vi "Start-Stop-Exp-Lock_UnLock.vi"(8 "entrée d'erreur (pas d'erreur)":errorcluster, 10 "Control-Client old entrée":refnum<class "Control-Client.lvclass">, 11 "Control-Client new entrée":refnum<class "Control-Client.lvclass">) -> (0 "sortie d'erreur":errorcluster, 2 "Control-Client old out":refnum<class "Control-Client.lvclass">, 3 "Control-Client new out":refnum<class "Control-Client.lvclass">)   [LabVIEW 2019, in "Control-Client.lvclass"]
uses:
  Control-Client.lvclass
  Control-Client.lvclass/Control-Client.ctl
  controls/Gauge_pump/Gauge_pump.xctl
  dependecies/XControls/CellsDL/ControlDL.xctl
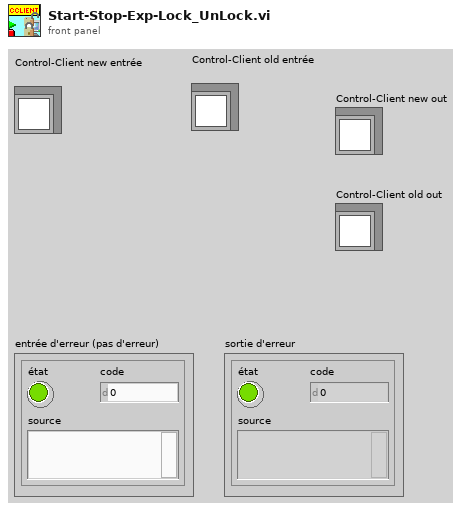
[diagram p1: front panel]
types:
  T1 = enum8{"Enabled", "Disabled", "Disabled and Grayed Out"}
  T2 = typedef "Control-Client.lvclass/Controls-with-permissions_CLIENT.ctl" = cluster{"Server ON/OFF":refnum<vi>, "Detector connect":refnum<vi>, "DL connect":refnum<vi>, "DAQmx connect":refnum<vi>, "All connect":refnum<vi>, "Start measurement":refnum<vi>, "Move Crystal":refnum<vi>, "Relay key heater":refnum<vi>, "Laser Shutter":refnum<vi>, "Accelerator Shutter":refnum<vi>, "Power":refnum<vi>, "Unlock":refnum<vi>, "RT":refnum<vi>, "Faraday Cup":refnum<vi>, "Osc connect":refnum<vi>, "ELYSE pulses":refnum<vi>, "Cells":refnum<vi>, "Pump":refnum<vi>, "# par point":refnum<vi>, "Alarm":refnum<vi>, "oscilloscopeRead":refnum<vi>, "WCM_state":refnum<vi>, "ControlDL":refnum<vi>}
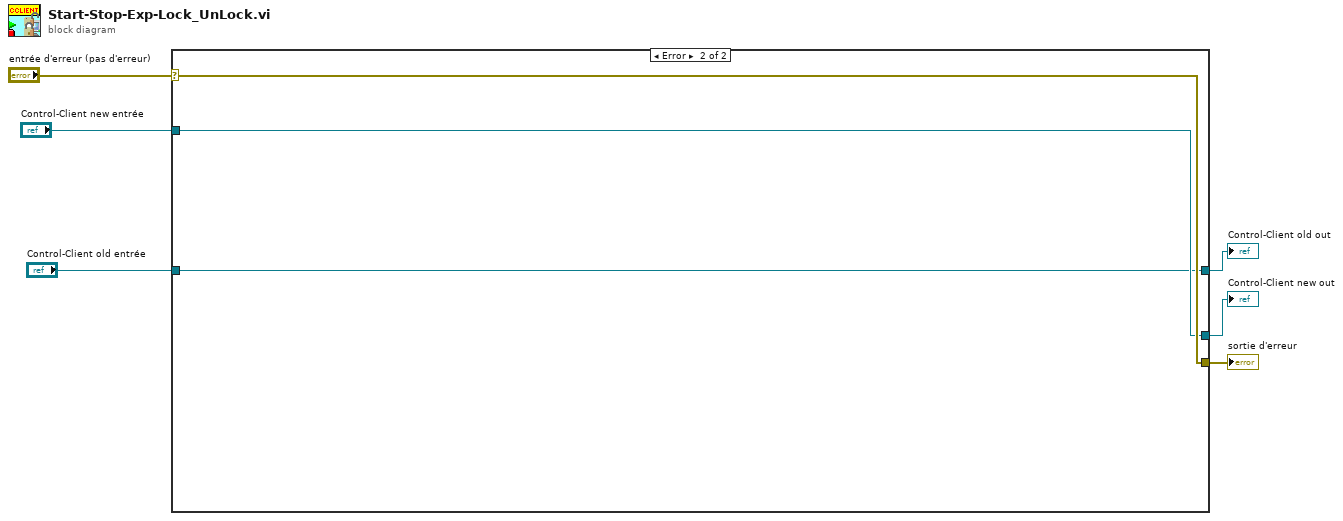
[diagram p0: block diagram]
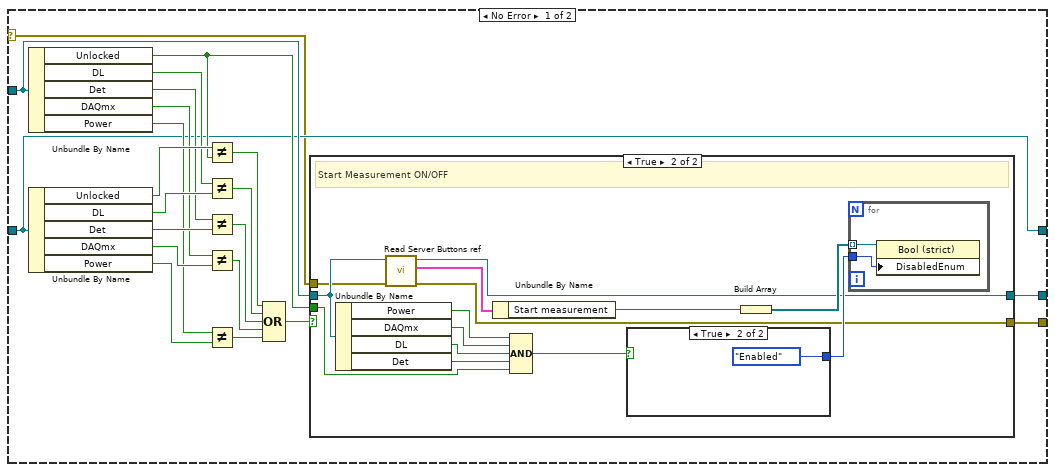
[diagram p2: hidden frame]
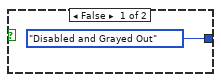
[diagram p4: hidden frame]
diagram:
  n1 = case shown="Error" "entrée d'erreur (pas d'erreur)" {
    selector: "entrée d'erreur (pas d'erreur)" -> [w7 w50]
    tunnel: [w27 w50] -> w6
    tunnel: "Control-Client new entrée" -> [w26 w49]
    tunnel: [w9 w49] -> w4
    tunnel: "Control-Client old entrée" -> [w8 w48]
    tunnel: [w8 w48] -> w1
    frame No Error {
      n2 = Unbundle By Name(w26) -> ("Unlocked"=w24:bool, "DL"=w23:bool, "Det"=w20:bool, "DAQmx"=w19:bool, "Power"=w16:bool)
      n3 = Unbundle By Name(w8) -> ("Unlocked"=w25:bool, "DL"=w22:bool, "Det"=w21:bool, "DAQmx"=w18:bool, "Power"=w17:bool)
      n4 = Not Equal?(x=w25, y=w24) -> (x != y?=w15:bool)
      n5 = Not Equal?(x=w23, y=w22) -> (x != y?=w14:bool)
      n6 = Not Equal?(x=w20, y=w21) -> (x != y?=w13:bool)
      n7 = Not Equal?(x=w19, y=w18) -> (x != y?=w11:bool)
      n8 = Not Equal?(x=w16, y=w17) -> (x != y?=w12:bool)
      n9 = Compound Arithmetic op=OR ("Opérateur arithmétique")(w15, w14, w13, w11, w12) -> (w10:bool)
      n10 = case shown="True" w10 {
        tunnel: w26 -> [w29 w36]
        tunnel: [w28 w39] -> w27
        tunnel: w24 -> [_ w38]
        tunnel: [w29 w31] -> w9
        tunnel: w7 -> [w28 w30]
        frame False {
        }
        frame True {
          # "Start Measurement ON/OFF"
          n11 = Unbundle By Name(w36) -> ("Power"=w32:bool, "DAQmx"=w35:bool, "DL"=w34:bool, "Det"=w33:bool)
          n12 = call "Read Server Buttons ref.vi"("error in (no error)"=w30, "Control-Client in"=w36) -> ("error out"=w39:errorcluster, "Server Buttons ref"=w43:T2, "Control-Client out"=w31:refnum<class "Control-Client.lvclass">)  [unwired: 7 in]
          n13 = Unbundle By Name(w43) -> ("Start measurement"=w42:refnum<vi>)
          n14 = Compound Arithmetic op=AND(w32, w35, w34, w33, w38) -> (w37:bool)
          n15 = case shown="True" w37 {
            tunnel: [T1."Disabled and Grayed Out" ("Désactivé") T1."Enabled" ("Désactivé")] -> w41
            frame False {
            }
            frame True {
            }
          }
          n16 = Build Array(w42) -> (w40:refnum<vi>[])
          n17 = for {
            tunnel: w40 -> [w47] mode=indexing
            tunnel: w41 -> [w46]
            n18 = property class="Bool (strict)"(reference=w47, "DisabledEnum"=w46) -> ()  [unwired: 1 in, 2 out]
          }
        }
      }
    }
    frame Error {
    }
  }
  "sortie d'erreur" <- w6
  "Control-Client new out" <- w4
  "Control-Client old out" <- w1
